vi "Do.vi"(8 "error in (no error)":errorcluster, 10 "Actor in":refnum<class "Actor.lvclass">, 11 "Scan Hardware Message":refnum<class "Scan Hardware Message.lvclass">) -> (0 "error out":errorcluster, 2 "Actor out":refnum<class "Actor.lvclass">)   [LabVIEW 2016, in "Controller Actor.lvlib" / "Scan Hardware Message.lvclass"]
uses:
  <userlib>/Common Components/Controller/Messages/Scan Hardware Message/Scan Hardware Message.lvclass
  <vilib>/ActorFramework/Actor/Actor.lvclass
  <userlib>/Common Components/Controller/Controller.lvclass
  C:/Program Files (x86)/National Instruments/LabVIEW 2016/vi.lib/ActorFramework/Actor/Actor.lvclass
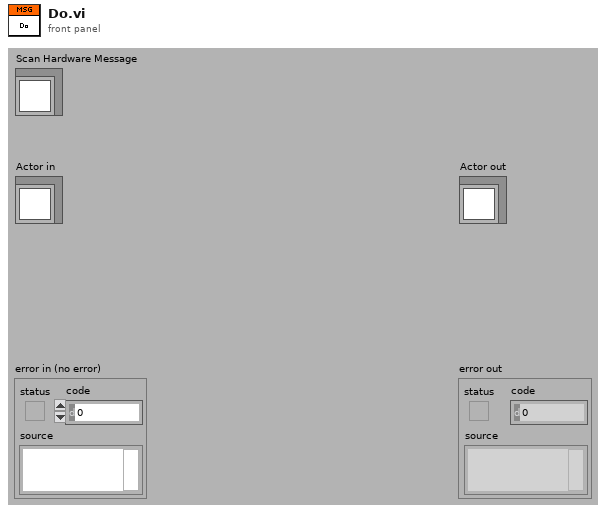
[diagram p1: front panel]
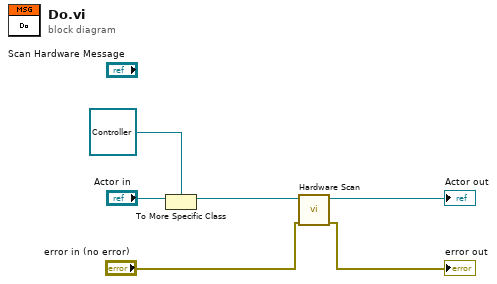
[diagram p0: block diagram]
diagram:
  n1 = To More Specific Class(target class=refnum<class "Controller.lvclass"> refnum ("Controller.lvclass"), reference="Actor in") -> (specific class reference=w4:refnum<class "Controller.lvclass">)  [unwired: 1 in, 1 out]
  n2 = call-dynamic "Hardware Scan.vi"("error in (no error)"="error in (no error)", "Controller in"=w4) -> ("error out"=→"error out":errorcluster, "Controller out"=→"Actor out":refnum<class "Controller.lvclass">)  [unwired: 8 in]
